vi "PathPlanner_PathFinder_SendCommand.vi"(8 "error in (no error)":errorcluster, 11 "PathFindingCommand":T1) -> (0 "error out":errorcluster)   [LabVIEW 2019, in "PathPlanner24.lvlib"]
doc: "Internal function. Not to be used by end users."
uses:
  PathPlanner24.lvlib
  ENum/PathPlanner_PathFinding_Cmd_ENUM.ctl
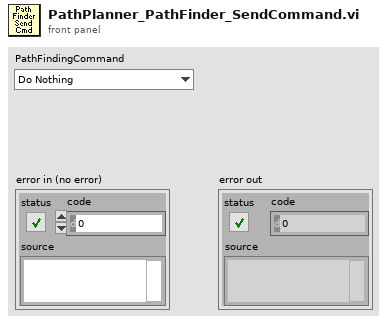
[diagram p1: front panel]
types:
  T1 = typedef "PathPlanner24.lvlib/PathPlanner_PathFinding_Cmd_ENUM.ctl" = enum16{"Do Nothing", "Reset", "Minor", "Reset and Minor", "Major", "Reset and Major", "Minor and Major", "Reset, Minor, Major"}
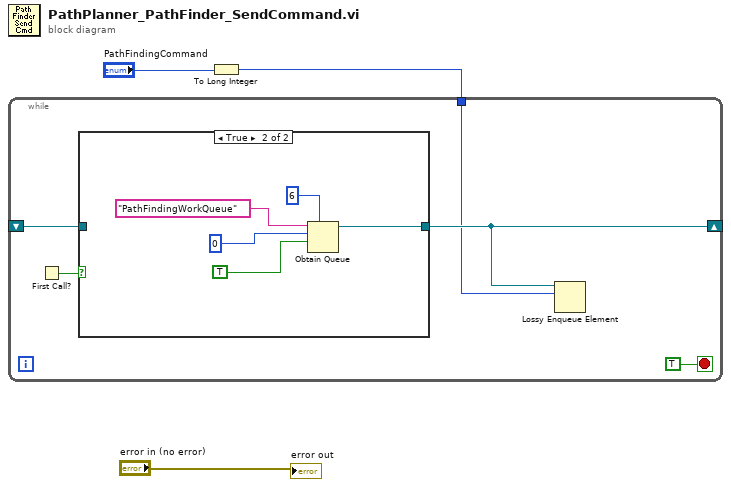
[diagram p0: block diagram]
diagram:
  n1 = To Long Integer(number="PathFindingCommand") -> (32bit integer=w2:i32)
  n2 = while {
    shift-right: [w6] -> _
    shift-left: _ -> [w5]
    tunnel: w2 -> [w4]
    stop <- TRUE stop-if-true
    n3 = First Call?() -> (First Call?: T/F=w7:bool)
    n4 = case shown="True" w7 {
      tunnel: [w9 w10] -> w6
      tunnel: w5 -> [w9 _]
      frame False {
      }
      frame True {
        n5 = Obtain Queue(max queue size (-1, unlimited)=6, name (unnamed)="PathFindingWorkQueue", element data type=0, create if not found? (T)=TRUE) -> (queue out=w10:refnum<queue>)  [unwired: 1 in, 2 out]
      }
    }
    n6 = Lossy Enqueue Element(queue=w6, element=w4) -> ()  [unwired: 1 in, 4 out]
  }
  "error out" <- "error in (no error)"
